vi "Delete Attribute.vi"(7 "Tree ID":string, 8 "Error In":errorcluster, 10 "Attribute Name":string, 11 "Tree Manager":T1) -> (0 "Error Out":errorcluster, 1 "Attribute Value":variant, 2 "Found?":bool, 3 "Tree Manager":T1)   [LabVIEW 2016, in "Tree Manager.lvclass"]
doc: "Delete a variant attribute from the Tree and return it."
uses:
  Tree Manager.lvclass
  Typedefs/Session Handle.ctl
  Tree Manager.lvclass/Tree Manager.ctl
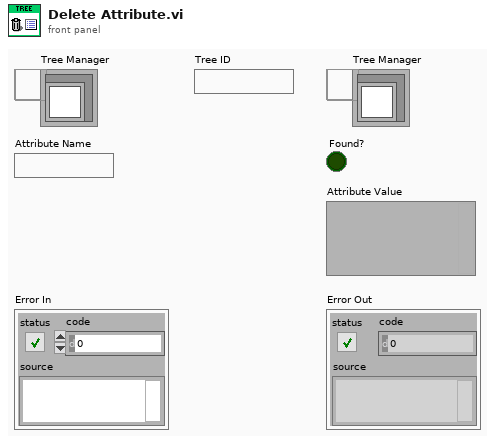
[diagram p1: front panel]
types:
  T1 = typedef "Tree Manager.lvclass/Session Handle.ctl" = refnum<data-value>
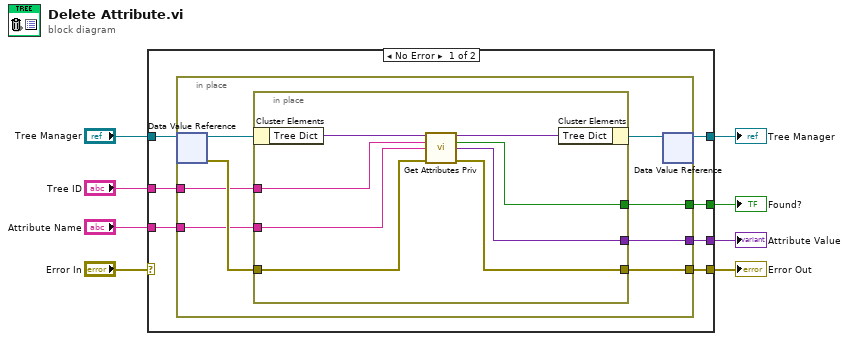
[diagram p0: block diagram]
diagram:
  n1 = case shown="No Error" "Error In" {
    selector: "Error In" -> [_ w32]
    tunnel: "Tree Manager" -> [w15 w33]
    tunnel: [w14 w33] -> w7
    tunnel: [w13 w32] -> w5
    tunnel: "Tree ID" -> [w12 _]
    tunnel: "Attribute Name" -> [w11 _]
    tunnel: [w10 _] -> w2
    tunnel: [w9 _] -> w1
    frame No Error {
      n2 = in-place {
        in-place-border: [w22] -> w13
        in-place-border: w12 -> [w19]
        in-place-border: w11 -> [w18]
        in-place-border: [w17] -> w10
        in-place-border: [w16] -> w9
        n3 = in-place-dvr #1(w15) -> (w23:refnum<class "Tree Manager.lvclass">, w20:errorcluster)
        n4 = in-place {
          in-place-border: [w24] -> w22
          in-place-border: w20 -> [w29]
          in-place-border: w19 -> [w28]
          in-place-border: w18 -> [w27]
          in-place-border: [w26] -> w17
          in-place-border: [w25] -> w16
          n5 = in-place-cluster #2(w23) -> ("Tree Dict"=w31:variant)
          n6 = call "Get Attributes Priv.vi"("Tree Dictionary In"=w31, "Unique ID"=w28, "Name"=w27, "error in"=w29) -> ("Tree Dictionary Out"=w30:variant, "Found?"=w26:bool, "Data"=w25:variant, "error out"=w24:errorcluster)  [unwired: 8 in]
          n7 = in-place-cluster #2("Tree Dict"=w30) -> (w21:refnum<class "Tree Manager.lvclass">)
        }
        n8 = in-place-dvr #1(w21) -> (w14:T1)  [unwired: 1 out]
      }
    }
    frame Error {
    }
  }
  "Tree Manager" <- w7
  "Error Out" <- w5
  "Found?" <- w2
  "Attribute Value" <- w1
